vi "Read timeouts.vi"(8 "error in (no error)":errorcluster, 11 "Master CR in":refnum<class "Master CR.lvclass">) -> (0 "error out":errorcluster, 2 "MB timeouts":T1={"reconn_timeout"=3000, "N attempt max"=3, "t_reset_TTL"=120000, "period"=100} {"t_reset_TTL" min=10 max=240000 step=1; "period" min=10 max=100000 step=1; "N attempt max" min=1 max=5 step=1; "reconn_timeout" min=10 max=240000 step=1}, 3 "Master CR out":refnum<class "Master CR.lvclass">)   [LabVIEW 2021, in "Master CR.lvclass"]
uses:
  Master CR.lvclass
  ctl/MB timeouts.ctl
  Master CR.lvclass/Master CR.ctl
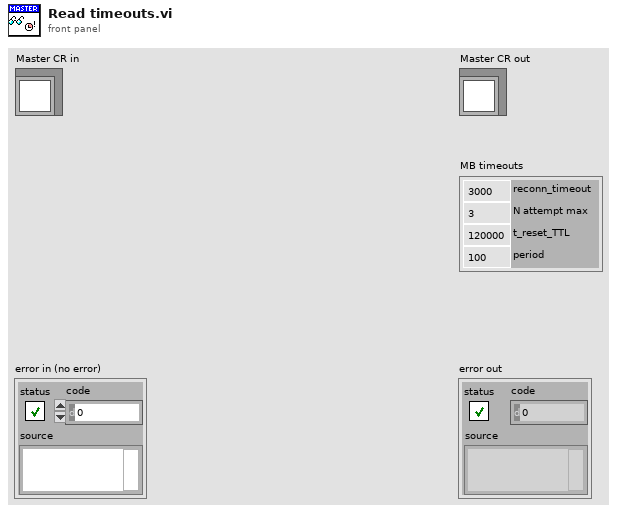
[diagram p1: front panel]
types:
  T1 = typedef "Master CR.lvclass/MB timeouts.ctl" = cluster{"reconn_timeout":i32, "N attempt max":i32, "t_reset_TTL":i32, "period":i32}
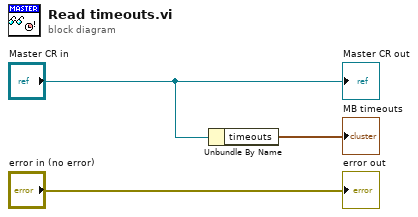
[diagram p0: block diagram]
diagram:
  n1 = Unbundle By Name("Master CR in") -> ("timeouts"=→"MB timeouts":T1)
  "error out" <- "error in (no error)"
  "Master CR out" <- "Master CR in"
